vi "Set Busy Element.vi"(7 "New Block":u32, 8 "error in (no error)":errorcluster, 10 "Indexes":cluster{"Row":i16, "Column":i16}, 11 "Board in":refnum<class "Board.lvclass">) -> (0 "error out":errorcluster, 3 "Board out":refnum<class "Board.lvclass">)   [LabVIEW 2017, in "Board.lvclass"]
uses:
  Board.lvclass
  Board.lvclass/Board.ctl
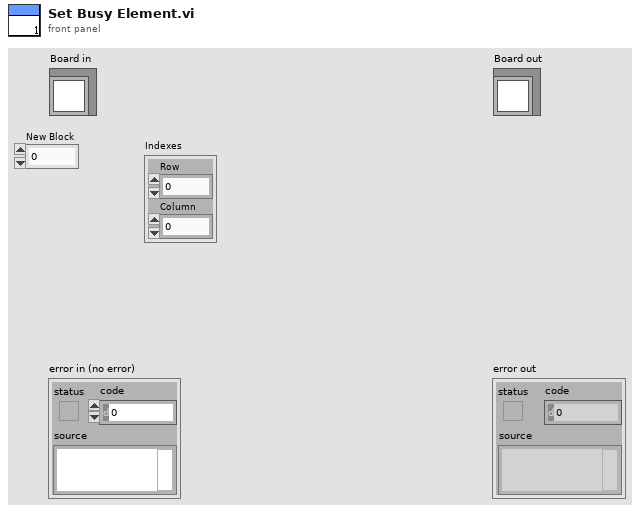
[diagram p1: front panel]
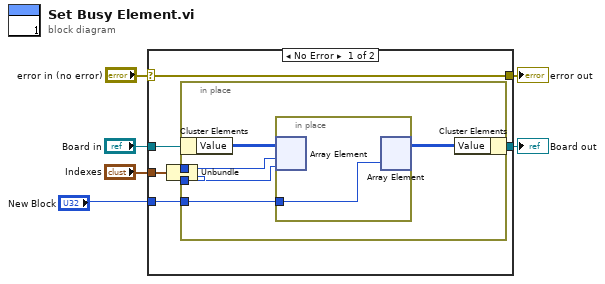
[diagram p0: block diagram]
diagram:
  n1 = case shown="No Error" "error in (no error)" {
    selector: "error in (no error)" -> [w13 w21]
    tunnel: [w13 w21] -> w5
    tunnel: [w11 w20] -> w3
    tunnel: "Board in" -> [w12 w20]
    tunnel: "Indexes" -> [w10 _]
    tunnel: "New Block" -> [w7 _]
    frame No Error {
      n2 = Unbundle(w10) -> ("Row"=w9:i16, "Column"=w8:i16)
      n3 = in-place {
        in-place-border: w9 -> [w17]
        in-place-border: w8 -> [w16]
        in-place-border: w7 -> [w14]
        n4 = in-place-cluster #1(w12) -> ("Value"=w18:u32[][])
        n5 = in-place {
          in-place-border: w14 -> [w19]
          n6 = in-place-array #2(w18, w17, w16) -> ()  [unwired: 1 out]
          n7 = in-place-array #2(w19) -> (w15:u32[][])  [unwired: 2 out]
        }
        n8 = in-place-cluster #1("Value"=w15) -> (w11:refnum<class "Board.lvclass">)
      }
    }
    frame Error {
    }
  }
  "error out" <- w5
  "Board out" <- w3
